vi "sub_wfm-filtering.vi"(11 "wfm in":waveform(dbl)) -> (1 "wfm out":waveform(dbl)(graph)={"t0"=timestamp(5.399999999999914e-07 s since 1904-01-01), "dt"=2e-08, "Y"=array[1084 elements]}, 2 "Array":dbl[](array[numeric]), 3 "DC value":dbl=0.5683932841328418 format="%.2f")   [LabVIEW 2021]
uses:
  ctrl/rw.ctl
  <vilib>/Waveform/WDTOps.llb/WDT Get Waveform Subset DBL.vi
  <vilib>/measure/madcrms.llb/Basic Averaged DC-RMS for 1 Chan.vi
  <vilib>/measure/NI_MAPro.lvlib
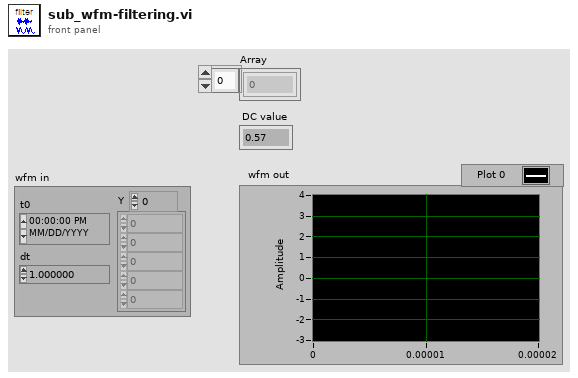
[diagram p1: front panel]
types:
  T1 = typedef "rw.ctl" = enum16{"read", "write"}
  T2 = typedef "wfm_cfg.ctl" = cluster{"history size":i32, "dim":i32, "start samples":dbl, "duration":dbl, "zeros":i32}
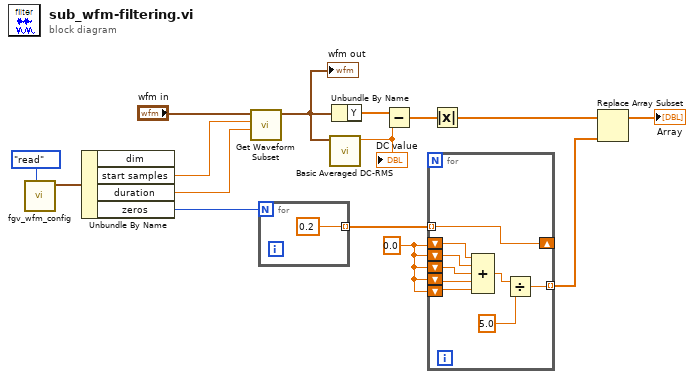
[diagram p0: block diagram]
diagram:
  w3 = 0.0
  n1 = call "fgv_wfm_config.vi"("cmd"=rw."read") -> ("wfm config 2"=w7:T2)  [unwired: 10 in]
  n2 = Unbundle By Name(w7) -> ("start samples"=w6:dbl, "duration"=w5:dbl, "zeros"=w4:i32)  [unwired: 1 out]
  n3 = call-poly <vilib>:"Get Waveform Subset.vi"("duration"=w5, "start samples/time"=w6, "waveform in"="wfm in") -> ("waveform out"=w9:waveform(dbl))  [unwired: 3 in, 3 out]
  "wfm out" <- w9
  n4 = for {
    N: w4 -> [_]
    tunnel: [0.2] -> w2 mode=indexing
  }
  n5 = call-poly <vilib>:"Basic Averaged DC-RMS.vi"("signal in"=w9) -> ("DC value"=w10:dbl)  [unwired: 7 in, 3 out]
  "DC value" <- w10
  n6 = Unbundle By Name(w9) -> ("Y"=w12:dbl[])
  n7 = Subtract(x=w12, y=w10) -> (x-y=w11:dbl[])
  n8 = for {
    tunnel: w2 -> [w25] mode=indexing
    shift-right: [w25] -> _
    shift-left: w3 -> [w21]
    shift-left: w3 -> [w22]
    shift-left: w3 -> [w23]
    shift-left: w3 -> [w24]
    tunnel: [w18] -> w1 mode=indexing
    shift-left: w3 -> [w17]
    n9 = Compound Arithmetic op=ADD(w21, w22, w23, w24, w17) -> (w20:dbl)
    n10 = Divide(x=w20, y=5.0) -> (x/y=w18:dbl)
  }
  n11 = Absolute Value(x=w11) -> (abs(x)=w13:dbl[])
  n12 = Replace Array Subset(array=w13, new element=w1) -> (→"Array":dbl[])  [unwired: 1 in]
